vi "Chart Range.vi"(8 "error in (no error)":errorcluster, 11 "HistorianCharting in":refnum<class "HistorianCharting.lvclass">) -> (0 "error out":errorcluster, 1 "End":dbl, 2 "Start":dbl, 3 "HistorianCharting out":refnum<class "HistorianCharting.lvclass">, 4 "Set Time":bool)   [LabVIEW 2020, in "VolatusGUIElements.lvlib" / "HistorianCharting.lvclass"]
uses:
  HistorianCharting.lvclass
  HistorianCharting.lvclass/HistorianCharting.ctl
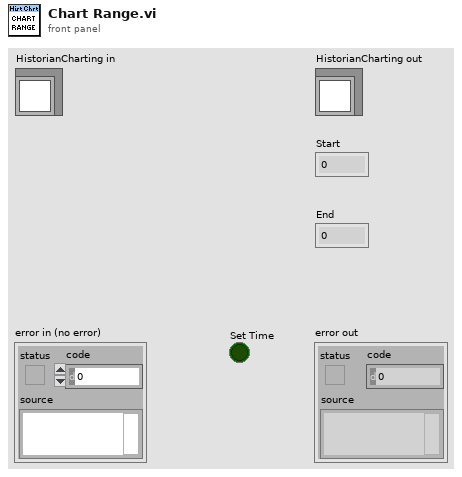
[diagram p1: front panel]
types:
  T1 = typedef "VolatusGUI.lvlib/Historian Charting Manager.lvclass/Plot Group Config.ctl" = cluster{"Name":string, "X-Axis Type":T2, "X-Axis Channel":string, "Plots":T3[], "Lock Now":bool, "Time":string, "Swap Axes":bool}
  T2 = typedef "VolatusGUI.lvlib/Historian Charting Manager.lvclass/X-Axis Type.ctl" = enum16{"Time", "Channel"}
  T3 = typedef "VolatusGUI.lvlib/Historian Charting Manager.lvclass/Plot Config.ctl" = cluster{"Channel":string, "Visible":bool, "Color":u32, "Scale":T4}
  T4 = typedef "VolatusGUI.lvlib/Historian Charting Manager.lvclass/Scale.ctl" = enum16{"Left", "Right"}
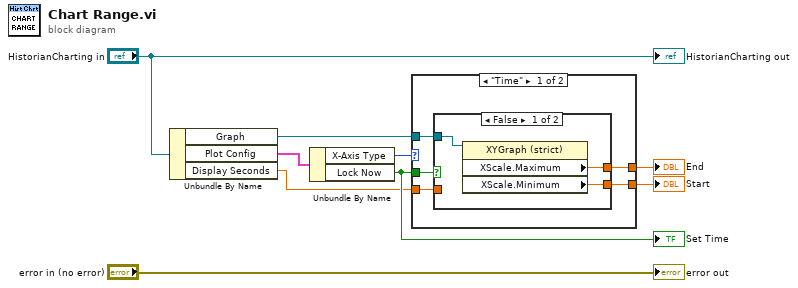
[diagram p0: block diagram]
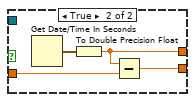
[diagram p2: hidden frame]
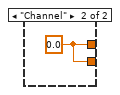
[diagram p3: hidden frame]
diagram:
  n1 = Unbundle By Name("HistorianCharting in") -> ("Graph"=w4:refnum<vi>, "Plot Config"=w8:T1, "Display Seconds"=w5:dbl)
  n2 = Unbundle By Name(w8) -> ("X-Axis Type"=w7:T2, "Lock Now"=w6:bool)
  "Set Time" <- w6
  n3 = case shown="\"Time\"" w7 {
    tunnel: w6 -> [w14 _]
    tunnel: w5 -> [w13 _]
    tunnel: [w12 w22] -> w2
    tunnel: [w11 w22] -> w1
    tunnel: w4 -> [w10 _]
    frame "Time" {
      n4 = case shown="False" w14 {
        tunnel: w13 -> [_ w20]
        tunnel: [w16 w18] -> w12
        tunnel: [w15 w19] -> w11
        tunnel: w10 -> [w17 _]
        frame False {
          n5 = property class="XYGraph (strict)"(reference=w17) -> ("XScale.Maximum"=w16:dbl, "XScale.Minimum"=w15:dbl)  [unwired: 1 in, 2 out]
        }
        frame True {
          n6 = Get Date/Time In Seconds() -> (seconds since 1Jan1904=w21:timestamp)
          n7 = To Double Precision Float(number=w21) -> (double precision float=w18:dbl)
          n8 = Subtract(x=w18, y=w20) -> (x-y=w19:dbl)
        }
      }
    }
    frame "Channel" {
      w22 = 0.0 ("XScale.Minimum")
    }
  }
  "Start" <- w1
  "End" <- w2
  "error out" <- "error in (no error)"
  "HistorianCharting out" <- "HistorianCharting in"
